vi "Read Functional Data (Single Correction).vi"(8 "error in (no error)":errorcluster, 11 "VISA resource name":refnum<visa-resource-name>) -> (0 "error out":errorcluster, 2 "Correction Data Array":dbl[](array[numeric]), 3 "VISA resource name out":refnum<visa-resource-name>)   [LabVIEW 2017, in "Agilent E4980.lvlib"]
doc: "Returns the open, short and load data for the single correction mode.\n\n<B>Notes:</B>\n(1) Returns 1,206 data for the 201 test points, even if you turn off some frequency points. If there is no correction data, the instrument returns 0.0.\n\n(2) Elements of the array are: <open1 A>,<open1 B>,<short1 A>,<short1 B>, <load1 A>,<load1 B>,<open2 A>,<open2 B>,<short2 A>,<short2 B>, <load2 A>,<load2 B>,....,<open201 A>,<open201 B>,<short201 A>, <short201 B>,<load201 A>,<load201 B>."
uses:
  Agilent E4980.lvlib
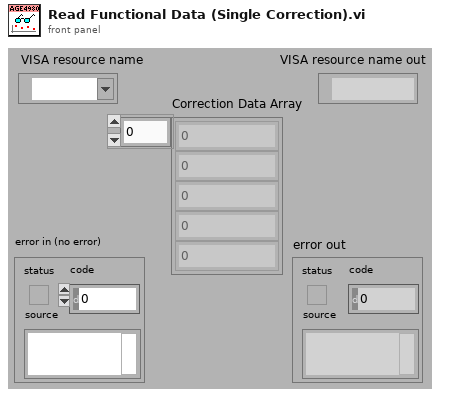
[diagram p1: front panel]
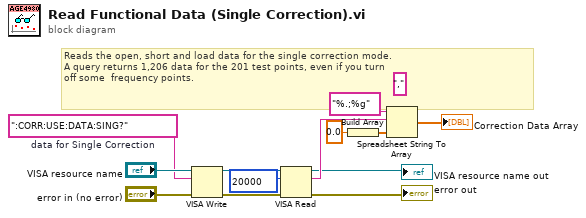
[diagram p0: block diagram]
diagram:
  w12 = ":CORR:USE:DATA:SING?"  # data for Single Correction
  # "Reads the open, short and load data for the single correction mode.\nA query returns 1,206 data for the 201 test points, even if you turn\noff some  frequency points."
  n1 = VISA Write(VISA resource name="VISA resource name", write buffer=w12, error in (no error)="error in (no error)") -> (VISA resource name out=w11:refnum<visa-resource-name>, error out=w10:errorcluster)  [unwired: 1 out]
  n2 = VISA Read(VISA resource name=w11, byte count=u32 20000, error in (no error)=w10) -> (VISA resource name out=→"VISA resource name out":refnum<visa-resource-name>, read buffer=w6:string, error out=→"error out":errorcluster)  [unwired: 1 out]
  n3 = Build Array(0.0) -> (w7:dbl[])
  n4 = Spreadsheet String To Array(delimiter (Tab)=",", format string="%.;%g", spreadsheet string=w6, array type (2D Dbl)=w7) -> (array=→"Correction Data Array":dbl[])
